vi "Updater Database Operations.vi"(6 "Debug (f)?":bool, 8 "error in (no error)":errorcluster, 11 "Spartan Install Path (empty)":path) -> (0 "error out":errorcluster, 1 "New Spartan":bool, 2 "Spartan Database Path":path, 3 "Connection Refnum":T1)   [LabVIEW 2011]
uses:
  Summitek EXT/ODBC/SQL Controls/Connection Refnum.ctl
  <vilib>/registry/registry.llb/Registry View.ctl
  <vilib>/registry/registry.llb/Read Registry Value Simple STR.vi
  Summitek EXT/OpenG EXT/file/file.llb/Valid Path - Traditional__ogtk.vi
  Summitek EXT/OpenG EXT/file/file.llb/File Exists - Scalar__ogtk.vi
  Summitek EXT/OpenG EXT/file/file.llb/Build Path - Traditional__ogtk.vi
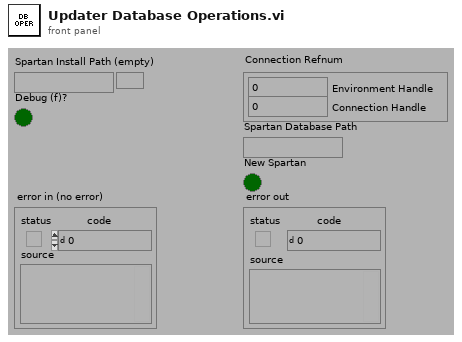
[diagram p1: front panel]
types:
  T1 = typedef "Connection Refnum.ctl" = cluster{"Environment Handle":i32, "Connection Handle":i32}
  T2 = typedef "Registry View.ctl" = u16
  T3 = typedef "Registry refnum.ctl" = refnum<k1>
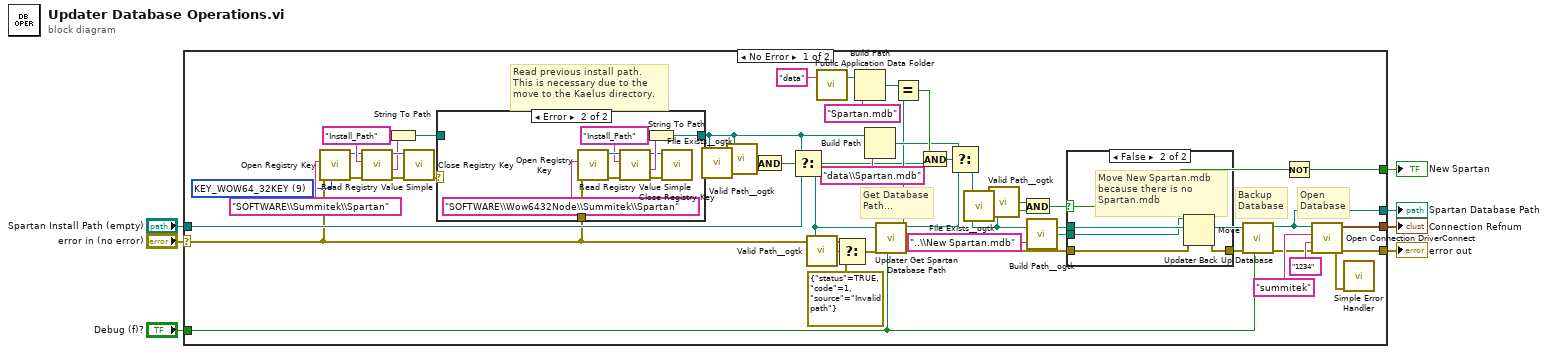
[diagram p0: block diagram]
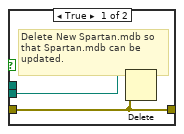
[diagram p3: hidden frame]
diagram:
  n1 = case shown="No Error" "error in (no error)" {
    selector: "error in (no error)" -> [w16 w69]
    tunnel: "Debug (f)?" -> [w47 _]
    tunnel: [w43 _] -> w6
    tunnel: [w42 _] -> w5
    tunnel: [w39 _] -> w4
    tunnel: "Spartan Install Path (empty)" -> [w31 _]
    tunnel: [w17 w69] -> w2
    frame No Error {
      w20 = T2 9 items=["Default"=0, "KEY_WOW64_64KEY"=8, "KEY_WOW64_32KEY"=9] ("registry view")
      # "Read previous install path.\nThis is necessary due to the\nmove to the Kaelus directory."
      # "Backup\nDatabase"
      # "Open\nDatabase"
      # "Get Database\nPath..."
      n2 = call <vilib>:"Open Registry Key.vi"("registry view"=w20, "error in (no error)"=w16, "subkey"="SOFTWARE\\Summitek\\Spartan") -> ("error out"=w32:errorcluster, "refnum out"=w33:T3)  [unwired: 7 in]
      n3 = call-poly <vilib>:"Read Registry Value Simple.vi"("error in (no error)"=w32, "value"="Install_Path" ("subkey"), "refnum"=w33) -> ("error out"=w36:errorcluster, "String/Binary data"=w35:string, "refnum out"=w37:T3)  [unwired: 3 in, 1 out]
      n4 = String To Path(string=w35) -> (path=w18:path)
      n5 = call <vilib>:"Close Registry Key.vi"("error in (no error)"=w36, "refnum"=w37) -> ("error out"=w19:errorcluster)  [unwired: 5 in]
      n6 = case shown="Error" w19 {
        tunnel: w18 -> [w53 _]
        tunnel: [w53 w54] -> w15
        tunnel: w16 -> [_ w55]
        frame No Error {
        }
        frame Error {
          n7 = call <vilib>:"Open Registry Key.vi"("error in (no error)"=w55, "subkey"="SOFTWARE\\Wow6432Node\\Summitek\\Spartan") -> ("error out"=w62:errorcluster, "refnum out"=w61:T3)  [unwired: 8 in]
          n8 = call-poly <vilib>:"Read Registry Value Simple.vi"("error in (no error)"=w62, "value"="Install_Path" ("subkey"), "refnum"=w61) -> ("error out"=w58:errorcluster, "String/Binary data"=w59:string, "refnum out"=w57:T3)  [unwired: 3 in, 1 out]
          n9 = String To Path(string=w59) -> (path=w54:path)
          n10 = call <vilib>:"Close Registry Key.vi"("error in (no error)"=w58, "refnum"=w57) -> ()  [unwired: 5 in, 1 out]
        }
      }
      n11 = call-poly "File Exists__ogtk.vi"("file path"=w15) -> ("exists"=w14:bool)  [unwired: 6 in, 1 out]
      n12 = call-poly "Valid Path__ogtk.vi"("path"=w15) -> ("valid"=w13:bool)
      n13 = And(x=w13, y=w14) -> (x .and. y?=w12:bool)
      n14 = Select(t=w15, s=w12, f=w31) -> (s? t:f=w30:path)
      n15 = call-poly "Valid Path__ogtk.vi"("path"=w30) -> ("valid"=w52:bool)
      n16 = call "Public Application Data Folder.vi"("Relative Path (\"\" - Folder)"="data" ("name or relative path")) -> ("Client Storage Path"=w27:path)  [unwired: 2 in]
      n17 = Select(t=w16, s=w52, f=errorcluster {"status"=TRUE, "code"=1, "source"="Invalid path"} ("error out")) -> (s? t:f=w50:errorcluster)
      n18 = Build Path(base path=w27, name or relative path="Spartan.mdb") -> (appended path=w26:path)
      n19 = Build Path(base path=w15, name or relative path="data\\Spartan.mdb") -> (appended path=w22:path)
      n20 = call "Updater Get Spartan Database Path.vi"("DEBUG? (f)"=w47, "error in (no error)"=w50, "Spartan Install Path (empty)"=w30) -> ("error out"=w45:errorcluster, "Spartan Database Path"=w21:path)  [unwired: 7 out]
      n21 = Equal?(x=w26, y=w21) -> (x = y?=w24:bool)
      n22 = And(x=w24, y=w12) -> (x .and. y?=w23:bool)
      n23 = Select(t=w22, s=w23, f=w21) -> (s? t:f=w9:path)
      n24 = call-poly "File Exists__ogtk.vi"("file path"=w9) -> ("exists"=w10:bool)  [unwired: 6 in, 1 out]
      n25 = call-poly "Valid Path__ogtk.vi"("path"=w9) -> ("valid"=w11:bool)
      n26 = And(x=w11, y=w10) -> (x .and. y?=w8:bool)
      n27 = call-poly "Build Path__ogtk.vi"("name or relative path"="..\\New Spartan.mdb", "base path"=w9) -> ("appended path"=w40:path)
      n28 = case shown="False" w8 {
        tunnel: w45 -> [w64 w67]
        tunnel: [w64 w66] -> w44
        tunnel: w9 -> [_ w68]
        tunnel: w40 -> [w63 w65]
        frame True {
          # "Delete New Spartan.mdb so\nthat Spartan.mdb can be\nupdated."
          n29 = Delete(path (use dialog)=w63, error in=w64) -> ()  [unwired: 3 in, 3 out]
        }
        frame False {
          # "Move New Spartan.mdb\nbecause there is no\nSpartan.mdb"
          n30 = Move(source path=w65, error in=w67, 10:w68) -> (error out=w66:errorcluster)  [unwired: 2 in, 2 out]
        }
      }
      n31 = call "Updater Back Up Database.vi"("DEBUG? (f)"=w47, "error in (no error)"=w44, "Database Path (empty)"=w9) -> ("error out"=w46:errorcluster, "dup Database Path"=w42:path)  [unwired: 7 out]
      n32 = Not(x=w8) -> (.not. x?=w39:bool)
      n33 = call "Open Connection DriverConnect.vi"("error in (no error)"=w46, "Password (\"\")"="1234" ("Username (\"\")"), "Username (\"\")"="summitek" ("Username (\"\")"), "ODBC Database (\"\")"=w42) -> ("error out"=w17:errorcluster, "Connection Refnum"=w43:T1)  [unwired: 3 out]
      n34 = call <vilib>:"Simple Error Handler.vi"("error in (no error)"=w17) -> ()  [unwired: 4 in, 5 out]
    }
    frame Error {
    }
  }
  "error out" <- w2
  "Connection Refnum" <- w6
  "Spartan Database Path" <- w5
  "New Spartan" <- w4
